vi "Write Top Level Values.vi"(8 "error in (no error)":errorcluster, 10 "Cluster of Top Level Values":variant, 11 "file path (use dialog)":path) -> (0 "error out":errorcluster)   [LabVIEW 2019, in "BlueTOMLSerializer.lvlib"]
uses:
  BlueTOMLSerializer.lvlib
  TOML Value.ctl
  TOML Key-Value Pair.ctl
  <vilib>/Utility/Data Type/NI_Data Type.lvlib
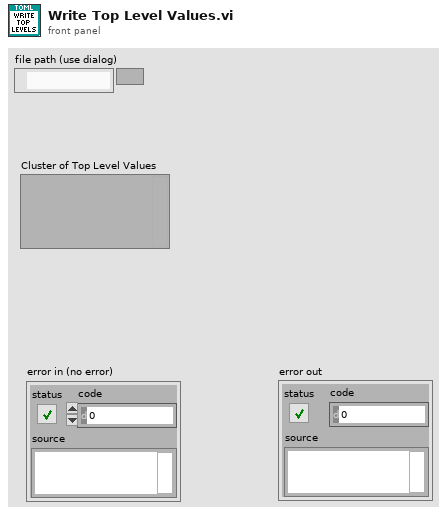
[diagram p1: front panel]
types:
  T1 = typedef "BlueTOMLSerializer.lvlib/TOML Key-Value Pair.ctl" = cluster{"Key":string, "Value":T2}
  T2 = typedef "BlueTOMLSerializer.lvlib/TOML Value.ctl" = cluster{"\\type":enum16{"Table", "Array", "String", "Integer", "Float", "Boolean", "Offset Date-Time", "Local Date-Time", "Local Date", "Local Time"}, "ÿýÿýÿýÿýÿýÿþÿýÿýÿý%LV-TOML.lvlib:TOML Key-Value Pair.ctlÿýÿýÿýÿýÿýÿþÿýÿýÿýLV-TOML.lvlib:TOML Value.ctl$":variant}
  T3 = enum16{"open", "replace", "create", "open or create", "replace or create", "replace or create with confirmation"}
  T4 = typedef "TOML.lvlib/TOML Value.ctl" = cluster{"\\type":enum16{"Table", "Array", "String", "Integer", "Float", "Boolean", "Offset Date-Time", "Local Date-Time", "Local Date", "Local Time"}, "ÿýÿýÿýÿýÿýÿþÿýÿýÿý%LV-TOML.lvlib:TOML Key-Value Pair.ctlÿýÿýÿýÿýÿýÿþÿýÿýÿýLV-TOML.lvlib:TOML Value.ctl$":variant}
  T5 = enum16{"Table", "Array", "String", "Integer", "Float", "Boolean", "Offset Date-Time", "Local Date-Time", "Local Date", "Local Time"}
  T6 = cluster{"\\type":enum16{"Table", "Array", "String", "Integer", "Float", "Boolean", "Offset Date-Time", "Local Date-Time", "Local Date", "Local Time"}, T1[]}
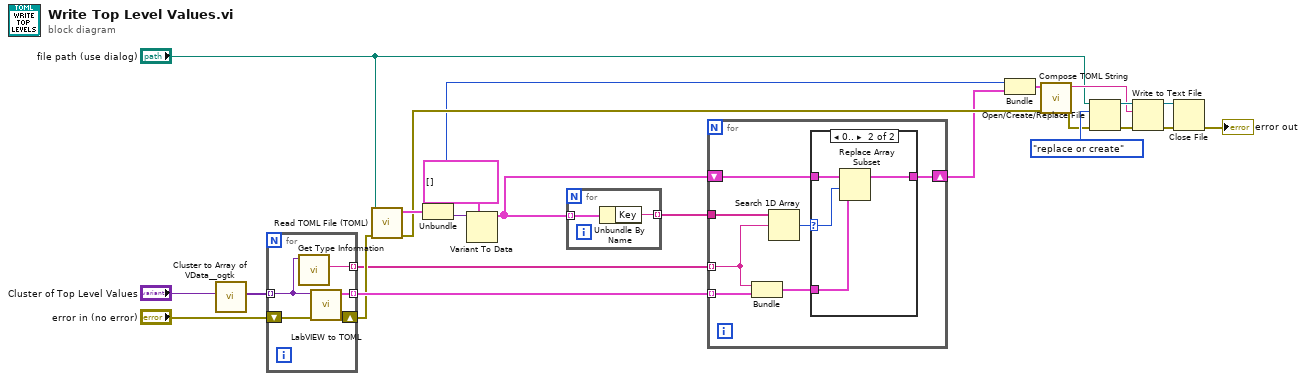
[diagram p0: block diagram]
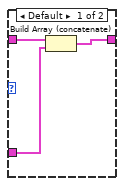
[diagram p2: hidden frame]
diagram:
  n1 = call <userlib>:"Cluster to Array of VData__ogtk.vi"("Cluster"="Cluster of Top Level Values") -> ("Array of VData"=w3:variant[])  [unwired: 9 in, 1 out]
  n2 = for {
    tunnel: [w27] -> w9 mode=indexing
    tunnel: w3 -> [w26] mode=indexing
    shift-right: [w28] -> w2
    shift-left: "error in (no error)" -> [w29]
    tunnel: [w25] -> w1 mode=indexing
    n3 = call <vilib>:"Get Type Information.vi"("variant"=w26) -> ("name"=w25:string)  [unwired: 6 in, 4 out]
    n4 = call "LabVIEW to TOML.vi"("error in (no error)"=w29, "LV Value"=w26) -> ("error out"=w28:errorcluster, "TOML Value"=w27:T4)  [unwired: 8 in]
  }
  n5 = call "Read TOML File (TOML).vi"("error in (no error)"=w2, "file path (use dialog)"="file path (use dialog)") -> ("error out"=w10:errorcluster, "Value"=w14:T2)  [unwired: 8 in]
  n6 = Unbundle(w14) -> ("\\type"=w7:T5, "ÿýÿýÿýÿýÿýÿþÿýÿýÿý%LV-TOML.lvlib:TOML Key-Value Pair.ctlÿýÿýÿýÿýÿýÿþÿýÿýÿýLV-TOML.lvlib:TOML Value.ctl$"=w13:variant)
  n7 = Variant To Data(type=T1[] [], Variant=w13) -> (data=w8:T1[])  [unwired: 1 in, 1 out]
  n8 = for {
    tunnel: w8 -> [w31] mode=indexing
    tunnel: [w30] -> w11 mode=indexing
    n9 = Unbundle By Name(w31) -> ("Key"=w30:string)
  }
  n10 = for {
    tunnel: w11 -> [w38]
    tunnel: w9 -> [w36] mode=indexing
    tunnel: w1 -> [w32] mode=indexing
    shift-right: [w33] -> w6
    shift-left: w8 -> [w34]
    n11 = Bundle("name"=w32, "TOML Value"=w36) -> (w35:cluster{"name":string, "TOML Value":T4})  [unwired: 1 in]
    n12 = Search 1D Array(1D array=w38, element=w32) -> (index of element=w37:i32)  [unwired: 1 in]
    n13 = case shown="0.." w37 {
      selector: w37 -> [_ w45]
      tunnel: w34 -> [w41 w42]
      tunnel: [w40 w44] -> w33
      tunnel: w35 -> [w39 w43]
      frame Default {
        n14 = Build Array (concatenate)(w41, w39) -> (w40:cluster{"name":string, "TOML Value":T4}[])
      }
      frame 0.. {
        n15 = Replace Array Subset(array=w42, new element=w43, index=w45) -> (w44:T1[])
      }
    }
  }
  n16 = Bundle("\\type"=w7, w6) -> (w5:T6)  [unwired: 1 in]
  n17 = call "Compose TOML String.vi"("error in (no error)"=w10, "Value"=w5) -> ("error out"=w16:errorcluster, "String"=w17:string)  [unwired: 8 in]
  n18 = Open/Create/Replace File(file path (use dialog)="file path (use dialog)", error in=w16, operation (0:open)=T3."replace or create") -> (refnum out=w22:refnum<file>, error out=w23:errorcluster)  [unwired: 3 in, 1 out]
  n19 = Write to Text File(file (use dialog)=w22, text=w17, error in=w23) -> (refnum out=w20:refnum<file>, error out=w21:errorcluster)  [unwired: 1 in, 1 out]
  n20 = Close File(refnum=w20, error in=w21) -> (error out=→"error out":errorcluster)  [unwired: 1 out]
